vi "SVE-Manager.vi"(9 "Data":variant, 10 "DataTag":string) -> (1 "error out":errorcluster)   [LabVIEW 2017]
uses:
  <vilib>/Utility/error.llb/DialogType.ctl
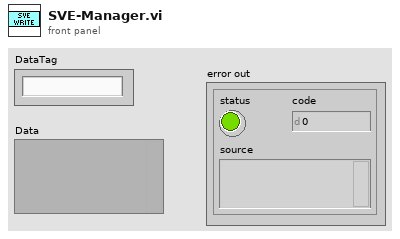
[diagram p1: front panel]
types:
  T1 = typedef "DialogType.ctl" = u16
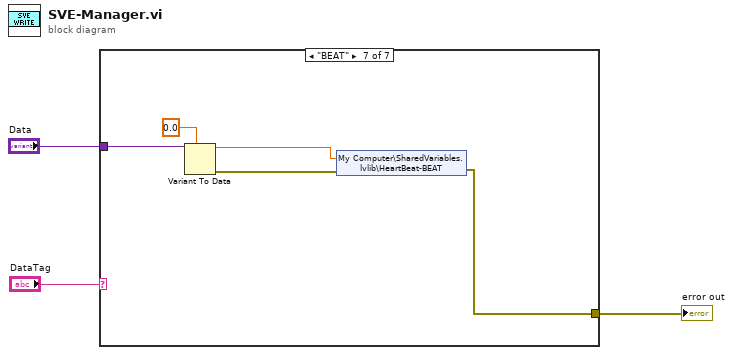
[diagram p0: block diagram]
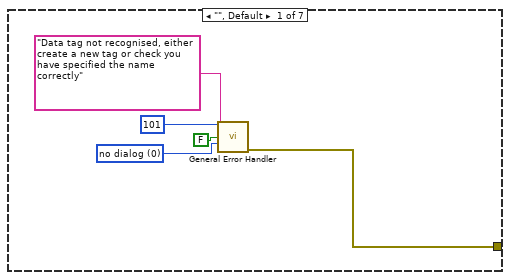
[diagram p2: hidden frame]
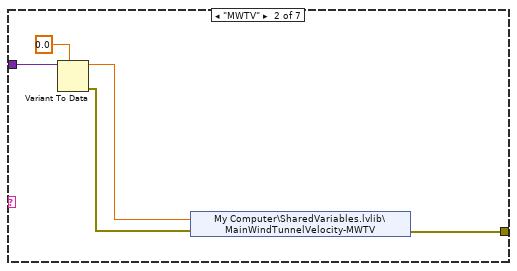
[diagram p3: hidden frame]
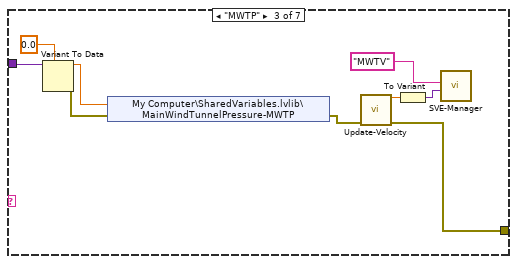
[diagram p4: hidden frame]
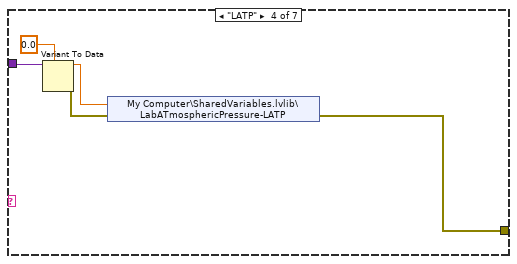
[diagram p5: hidden frame]
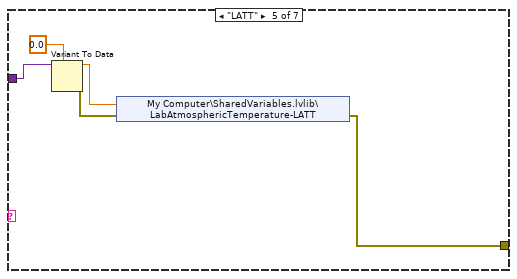
[diagram p6: hidden frame]
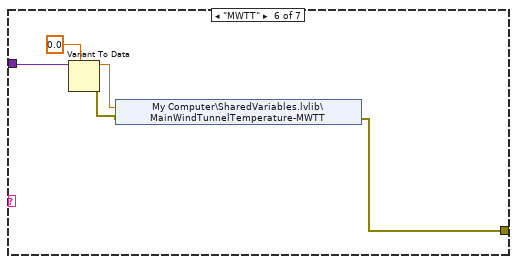
[diagram p7: hidden frame]
diagram:
  n1 = case shown="\"BEAT\"" "DataTag" {
    tunnel: [w8 w13 w15 w27 w28 w35 w39] -> w2
    tunnel: "Data" -> [_ w11 w21 w25 w29 w36 w41]
    frame "", Default {
      w6 = T1 0 items=["no dialog", "OK message", "continue or stop message", "OK message + warnings", "continue/stop + warnings"] ("type of dialog (OK msg:1)")
      n2 = call <vilib>:"General Error Handler.vi"("[error code] (0)"=101, "[error source] (\" \")"="Data tag not recognised, either create a new tag or check you have specified the name correctly" ("[error source] (\" \")"), "search ni.com link visible?(T)"=FALSE, "type of dialog (OK msg:1)"=w6) -> ("error out"=w8:errorcluster)  [unwired: 7 in, 4 out]
    }
    frame "MWTV" {
      n3 = Variant To Data(type=0.0 ("MainWindTunnelVelocity-MWTV"), Variant=w11) -> (data=w10:dbl, error out=w9:errorcluster)  [unwired: 1 in]
      n4 = shared-variable "My Computer\\SharedVariables.lvlib\\MainWindTunnelVelocity-MWTV"(w10, error in=w9) -> (error out=w13:errorcluster)
    }
    frame "MWTP" {
      n5 = Variant To Data(type=0.0 ("MainWindTunnelVelocity-MWTV"), Variant=w21) -> (data=w17:dbl, error out=w20:errorcluster)  [unwired: 1 in]
      n6 = shared-variable "My Computer\\SharedVariables.lvlib\\MainWindTunnelPressure-MWTP"(w17, error in=w20) -> (error out=w16:errorcluster)
      n7 = call "Update-Velocity.vi"("Error In"=w16) -> ("Error Out"=w15:errorcluster, "Velocity"=w14:dbl)  [unwired: 9 in]
      n8 = To Variant(anything=w14) -> (Variant=w18:variant)
      n9 = call "SVE-Manager.vi"("Data"=w18, "DataTag"="MWTV") -> ()  [unwired: 9 in, 1 out]
    }
    frame "LATP" {
      n10 = Variant To Data(type=0.0 ("MainWindTunnelVelocity-MWTV"), Variant=w25) -> (data=w23:dbl, error out=w24:errorcluster)  [unwired: 1 in]
      n11 = shared-variable "My Computer\\SharedVariables.lvlib\\LabATmosphericPressure-LATP"(w23, error in=w24) -> (error out=w27:errorcluster)
    }
    frame "LATT" {
      n12 = Variant To Data(type=0.0 ("MainWindTunnelVelocity-MWTV"), Variant=w29) -> (data=w31:dbl, error out=w32:errorcluster)  [unwired: 1 in]
      n13 = shared-variable "My Computer\\SharedVariables.lvlib\\LabAtmosphericTemperature-LATT"(w31, error in=w32) -> (error out=w28:errorcluster)
    }
    frame "MWTT" {
      n14 = Variant To Data(type=0.0 ("MainWindTunnelVelocity-MWTV"), Variant=w36) -> (data=w33:dbl, error out=w34:errorcluster)  [unwired: 1 in]
      n15 = shared-variable "My Computer\\SharedVariables.lvlib\\MainWindTunnelTemperature-MWTT"(w33, error in=w34) -> (error out=w35:errorcluster)
    }
    frame "BEAT" {
      n16 = Variant To Data(type=0.0 ("MainWindTunnelVelocity-MWTV"), Variant=w41) -> (data=w38:dbl, error out=w40:errorcluster)  [unwired: 1 in]
      n17 = shared-variable "My Computer\\SharedVariables.lvlib\\HeartBeat-BEAT"(w38, error in=w40) -> (error out=w39:errorcluster)
    }
  }
  "error out" <- w2
